vi "Get Default DV.vi"(8 "error in (no error)":errorcluster) -> (0 "error out":errorcluster, 3 "DV Default Value":i32)   [LabVIEW 2015]
uses:
  <vilib>/xml/Load XML File.vi
  <vilib>/xml/Close Reference(Node).vi
  <resource>/objmgr/DOMUserDefRef.rc
  <vilib>/xml/NI_XML.lvlib
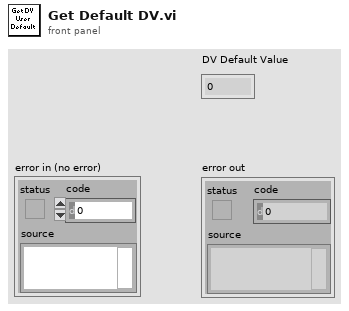
[diagram p1: front panel]
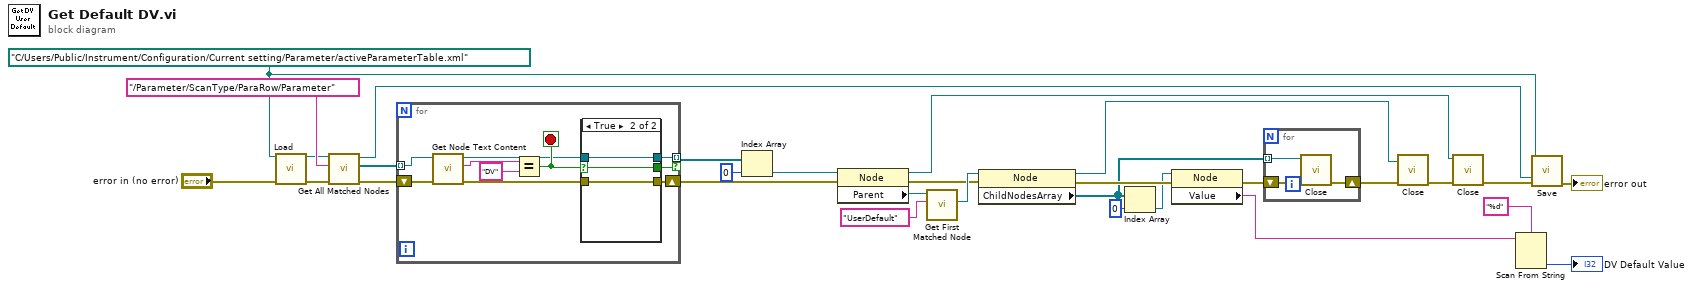
[diagram p0: block diagram]
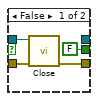
[diagram p2: hidden frame]
diagram:
  w25 = path "C:/Users/Public/Instrument/Configuration/Current setting/Parameter/activeParameterTable.xml" ("Load File")
  n1 = call-poly <vilib>:"Load.vi"("path to XML document"=w25, "error in (no error)"="error in (no error)") -> ("DOM document out"=w23:refnum<k20>, "error out"=w22:errorcluster)  [unwired: 11 in, 1 out]
  n2 = call <vilib>:"Get All Matched Nodes.vi"("error in (no error)"=w22, "XPath expression"="/Parameter/ScanType/ParaRow/Parameter" ("XPath Expression"), "node in"=w23) -> ("error out"=w29:errorcluster, "node result array"=w28:refnum<k20>[], "node out"=w27:refnum<k20>)  [unwired: 6 out]
  n3 = for {
    tunnel: w28 -> [w39] mode=indexing
    shift-right: [w35] -> w24
    shift-left: w29 -> [w40]
    tunnel: [w32] -> w7 mode=indexing if=w31
    stop <- w34 stop-if-true
    n4 = call <vilib>:"Get Node Text Content.vi"("error in (no error)"=w40, "node in"=w39) -> ("error out"=w36:errorcluster, "node text"=w37:string, "node out"=w33:refnum<k20>)  [unwired: 7 in]
    n5 = Equal?(x=w37, y="DV") -> (x = y?=w34:bool)
    n6 = case shown="True" w34 {
      selector: w34 -> [_ w45]
      tunnel: w36 -> [w44 w47]
      tunnel: [w43 w47] -> w35
      tunnel: w33 -> [w42 w46]
      tunnel: [_ w46] -> w32
      tunnel: [FALSE w45] -> w31
      frame False {
        n7 = call-poly <vilib>:"Close.vi"("error in (no error)"=w44, "node"=w42) -> ("error out"=w43:errorcluster)  [unwired: 7 in]
      }
      frame True {
      }
    }
  }
  n8 = Index Array(array=w7, index=0) -> (element=w9:refnum<k20>)
  n9 = property class="Node"(reference=w9, error in=w24) -> (reference out=w17:refnum<k20>, error out=w11:errorcluster, "Parent"=w14:refnum<k20>)
  n10 = call <vilib>:"Get First Matched Node.vi"("XPath expression"="UserDefault", "node in"=w14) -> ("node result"=w12:refnum<k20>)  [unwired: 7 in, 2 out]
  n11 = property class="Node"(reference=w12, error in=w11) -> (reference out=w21:refnum<k20>, error out=w10:errorcluster, "ChildNodesArray"=w5:refnum<k20>[])
  n12 = Index Array(array=w5, index=0) -> (element=w4:refnum<k20>)
  n13 = property class="Node"(reference=w4, error in=w10) -> (error out=w26:errorcluster, "Value"=w3:string)  [unwired: 1 out]
  n14 = for {
    shift-right: [w49] -> w20
    shift-left: w26 -> [w50]
    tunnel: w5 -> [w48] mode=indexing
    n15 = call-poly <vilib>:"Close.vi"("error in (no error)"=w50, "node"=w48) -> ("error out"=w49:errorcluster)  [unwired: 7 in]
  }
  n16 = call-poly <vilib>:"Close.vi"("error in (no error)"=w20, "node"=w21) -> ("error out"=w19:errorcluster)  [unwired: 7 in]
  n17 = call-poly <vilib>:"Close.vi"("error in (no error)"=w19, "node"=w17) -> ("error out"=w18:errorcluster)  [unwired: 7 in]
  n18 = Scan From String(format string="%d", input string=w3) -> (output 1=→"DV Default Value":i32)  [unwired: 3 in, 3 out]
  n19 = call <vilib>:"Save.vi"("error in (no error)"=w18, "XML file path"=w25, "DOM document in"=w27) -> ("error out"=→"error out":errorcluster)  [unwired: 6 in, 2 out]
